vi "IntakeStop.vi"   [LabVIEW 2014, in "IntakeLib.lvlib"]
uses:
  IntakeLib.lvlib
  <vilib>/Rock Robotics/WPI/Solenoid/WPI_SolenoidValue.ctl
types:
  T1 = typedef "WPI_SolenoidValue.ctl" = enum16{"Off", "On", "Forward", "Reverse"}
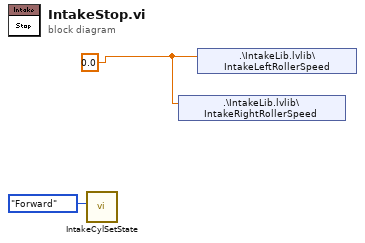
[diagram p0: block diagram]
diagram:
  w2 = 0.0
  n1 = call "IntakeCylSetState.vi"("IntakeCylState"=WPI_SolenoidValue."Forward") -> ()  [unwired: 11 in]
  n2 = shared-variable ".\\IntakeLib.lvlib\\IntakeRightRollerSpeed"(w2) -> ()  [unwired: 1 in, 1 out]
  n3 = shared-variable ".\\IntakeLib.lvlib\\IntakeLeftRollerSpeed"(w2) -> ()  [unwired: 1 in, 1 out]
